vi "Read Scan Configuration.vi"(8 "error in (no error)":errorcluster, 11 "Keithley 622x2182 Driver in":refnum<class "Keithley 622x2182 Driver.lvclass">) -> (0 "error out":errorcluster, 2 "Configuration":T1={"Start"=-0.001, "End"=0.001, "Step"=0.0001, "Scan shape"=enum."Sawtooth", "Append measurements"=[]} {"Step" format="%#_6p"; "End" format="%#_6p"; "Start" format="%#_6p"}, 3 "Keithley 622x2182 Driver out":refnum<class "Keithley 622x2182 Driver.lvclass">)   [LabVIEW 2021, in "Keithley 622x2182 Driver.lvclass"]
uses:
  Keithley 622x2182 Driver.lvclass
  Keithley 622x2182 Driver.lvclass/Keithley 622x2182 Driver.ctl
  Controls/Stepper Config.ctl
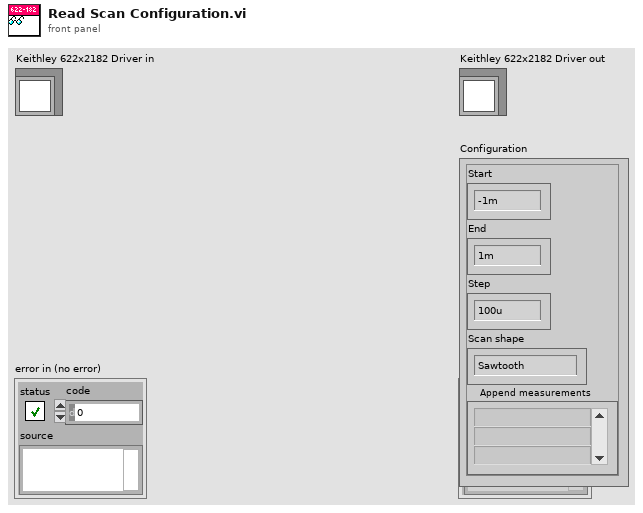
[diagram p1: front panel]
types:
  T1 = typedef "Stepper Config.ctl" = cluster{"Start":dbl, "End":dbl, "Step":dbl, "Scan shape":enum16{"Sawtooth", "Triangular"}, "Append measurements":string[]}
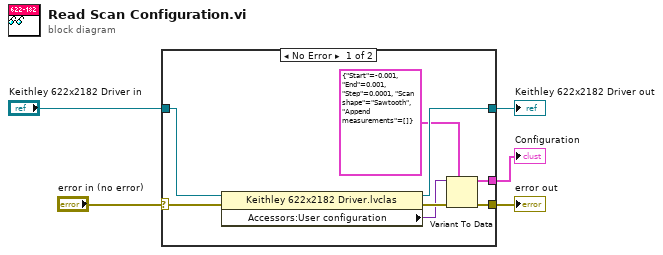
[diagram p0: block diagram]
diagram:
  n1 = case shown="No Error" "error in (no error)" {
    selector: "error in (no error)" -> [w13 w14]
    tunnel: [w9 w14] -> w4
    tunnel: [w11 w15] -> w2
    tunnel: "Keithley 622x2182 Driver in" -> [w12 w15]
    tunnel: [w6 _] -> w1
    frame No Error {
      n2 = property class="Keithley 622x2182 Driver.lvclas"(reference=w12, error in=w13) -> (reference out=w11:refnum<class "Keithley 622x2182 Driver.lvclass">, error out=w10:errorcluster, "Accessors:User configuration"=w8:variant)
      n3 = Variant To Data(error in=w10, type=T1 {"Start"=-0.001, "End"=0.001, "Step"=0.0001, "Scan shape"=enum."Sawtooth", "Append measurements"=[]} ("Scan Configuration"), Variant=w8) -> (data=w6:T1, error out=w9:errorcluster)
    }
    frame Error {
    }
  }
  "error out" <- w4
  "Keithley 622x2182 Driver out" <- w2
  "Configuration" <- w1
